vi "test.ingest_parquet 2.vi"   [LabVIEW 2020]
uses:
  datasources/dataset/dataset.lvclass
  nominal types/channelConfig/channelConfig.lvclass
  Nominal Client/Nominal Client.lvclass/Nominal Client.ctl
  nominal types/workspace/workspace.lvclass/workspace.ctl
  f68fde30-30e4-4b08-97bf-6f7da0132bc9.vi
  d999190f-fee9-49b3-afb9-f232f2b660b8.vi
  Nominal Client/private_data.set.vi
  nominal types/workspace/id.get.vi
  nominal types/workspace/rid.get.vi
  <vilib>/AdvancedString/1D String Array to Delimited String.vi
  Nominal Client/workspace.set.vi
  datasources/s3/s3.lvclass
  C:/code/labview-client/lv_src/datasources/source/source.lvclass
  <vilib>/Utility/error.llb/Error Cluster From Error Code.vi
  Nominal Client/workspace_cache.get_from_rid.vi
  Nominal Client/workspace_cache.get.vi
  ts.iso8601/build.iso8601.vi
  datasources/target/create_new.vi
  datasources/source/create_s3.vi
  Nominal Client/ingest_parquet.vi
  Nominal Client/Nominal Client.lvclass
  nominal types/workspace/workspace.lvclass
  submodules/reqwest-labview/lv-src/reqwest/reqwest.lvclass
  timestampMetadata/timestampMetadata.lvclass
  datasources/source/source.lvclass
  datasources/target/target.lvclass
  ts.iso8601/ts.iso8601.lvclass
  nominal types/properties/properties.lvclass
  C:/code/labview-client/lv_src/datasources/payload/payload.lvclass
  C:/code/labview-client/lv_src/datasources/s3/s3.lvclass
types:
  T1 = cluster{"dataset":refnum<class "dataset.lvclass">, "channelConfig":refnum<class "channelConfig.lvclass">}
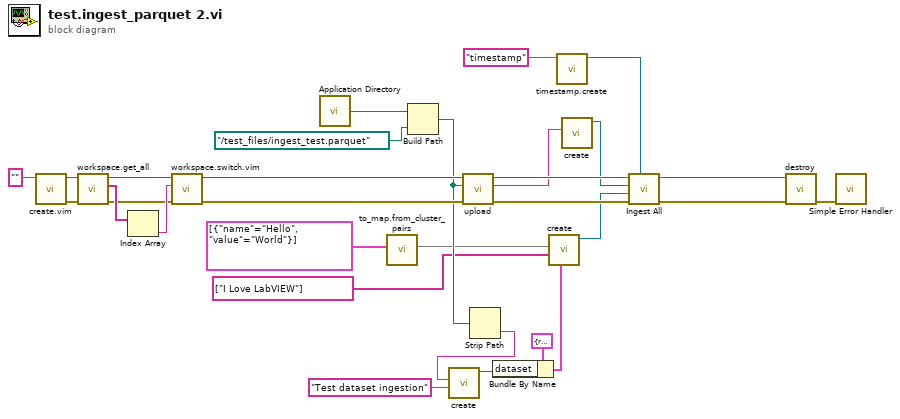
[diagram p0: block diagram]
diagram:
  n1 = call "create.vim"("API Token (string or path)"="") -> ("error out"=w15:errorcluster, "Nominal Client"=w19:refnum<class "Nominal Client.lvclass">)  [unwired: 9 in]
  n2 = call "workspace.get_all.vi"("error in"=w15, "Nominal Client in"=w19) -> ("error out"=w14:errorcluster, "Workspace RIDs"=w17:string[], "Nominal Client out"=w18:refnum<class "Nominal Client.lvclass">)  [unwired: 5 in, 2 out]
  n3 = Index Array(array=w17) -> (element=w16:string)  [unwired: 1 in]
  n4 = call "workspace.switch.vim"("error in"=w14, "Workspace RID (string or path)"=w16, "Nominal Client in"=w18) -> ("error out"=w13:errorcluster, "Nominal Client out"=w12:refnum<class "Nominal Client.lvclass">)  [unwired: 7 in]
  n5 = call <vilib>:"Application Directory.vi"() -> ("Application Directory"=w22:path)
  n6 = call "to_map.from_cluster_pairs.vi"("properties (cluster pairs)"=cluster{"name":string, "value":string}[] [{"name"="Hello", "value"="World"}] ("properties")) -> ("properties (map)"=w1:map{string, string})  [unwired: 10 in]
  n7 = Build Path(base path=w22, name or relative path=path "../test_files/ingest_test.parquet") -> (appended path=w6:path)
  n8 = call "upload.vi"("error in"=w13, "File"=w6, "Nominal Client in"=w12) -> ("error out"=w27:errorcluster, "Path to S3 File"=w26:string, "Nominal Client out"=w28:refnum<class "Nominal Client.lvclass">)  [unwired: 6 in]
  n9 = Strip Path(path=w6) -> (name=w5:string)  [unwired: 1 out]
  n10 = call "create.vi"("Description"="Test dataset ingestion", "Name"=w5) -> ("dataset"=w9:refnum<class "dataset.lvclass">)  [unwired: 9 in]
  n11 = Bundle By Name(cluster=T1 {"dataset"=refnum, "channelConfig"=refnum} ("Optional"), "dataset"=w9) -> (w10:T1)
  n12 = call-poly "create.vi"("Optional"=w10, "Labels"=string[] ["I Love LabVIEW"] ("labels"), "Properties"=w1) -> ("New Target"=w24:refnum<class "target.lvclass">)  [unwired: 8 in]
  n13 = call-poly "timestamp.create.vi"("seriesName"="timestamp") -> ("Timestamp Metadata"=w3:refnum<class "timestampMetadata.lvclass">)  [unwired: 10 in]
  n14 = call-poly "create.vi"("Path"=w26) -> ("source"=w25:refnum<class "s3.lvclass">)  [unwired: 10 in]
  n15 = call-poly "Ingest All.vi"("Timestamp Metadata"=w3, "error in"=w27, "Target"=w24, "Source"=w25, "Nominal Client in"=w28) -> ("error out"=w29:errorcluster, "Nominal Client out"=w30:refnum<class "Nominal Client.lvclass">)  [unwired: 3 in, 2 out]
  n16 = call "destroy.vi"("error in"=w29, "Nominal Client"=w30) -> ("error out"=w7:errorcluster)  [unwired: 9 in]
  n17 = call <vilib>:"Simple Error Handler.vi"("error in (no error)"=w7) -> ()  [unwired: 4 in, 5 out]
